vi "Get Magnet Field.vi"(6 "Axis":T1, 8 "error in (no error)":errorcluster, 11 "Instrument.Oxford1820 in":refnum<class "Instrument.Oxford1820.lvclass">) -> (0 "error out":errorcluster, 1 "Status":variant, 2 "B Field (T)":dbl, 3 "Instrument.Oxford1820 out":refnum<class "Instrument.Oxford1820.lvclass">, 4 "Finished?":bool)   [LabVIEW 2016, in "Instrument.Oxford1820.lvclass"]
uses:
  Instrument.Oxford1820.lvclass
  <userlib>/LevyLab/Levylab Instruments/Instrument Types/Cryostat/Typedefs/Magnet Axis--Enum.ctl
  Typedefs/Instrument.Oxford1820.Commands-enum.ctl
  <userlib>/LevyLab/Levylab Instruments/Instrument Types/Cryostat/Instrument.Cryostat.lvclass
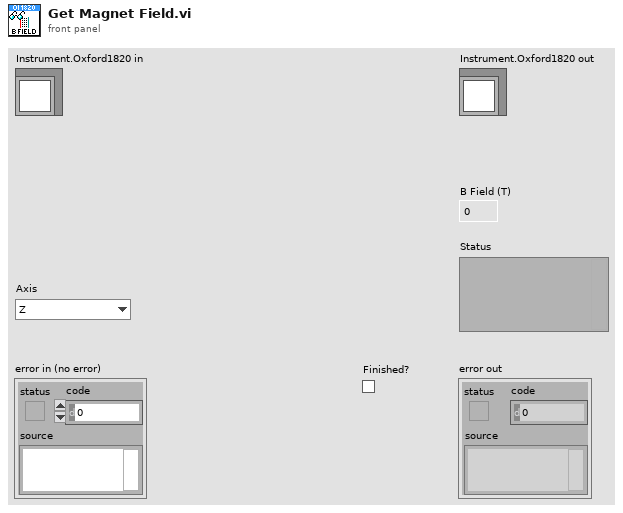
[diagram p1: front panel]
types:
  T1 = typedef "Instrument.Cryostat.lvclass/Magnet Axis--Enum.ctl" = enum16{"Z", "X", "Y"}
  T2 = typedef "Instrument.Oxford1820.lvclass/Instrument.Oxford1820.Commands-enum.ctl" = enum16{"setAction", "setTarget", "setSwitchHeat", "setLambda", "setFillMode", "setNeedleValve", "setMagnetField", "getStatus", "getTarget", "getSwitchHeat", "getPSUField", "newcommand", "getMagnetField"}
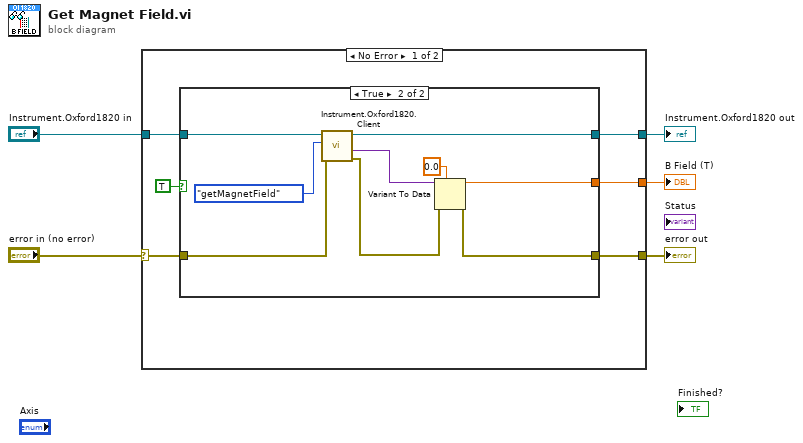
[diagram p0: block diagram]
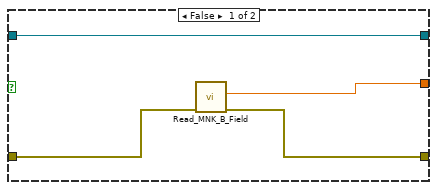
[diagram p2: hidden frame]
diagram:
  n1 = case shown="No Error" "error in (no error)" {
    selector: "error in (no error)" -> [w9 w26]
    tunnel: "Instrument.Oxford1820 in" -> [w7 w25]
    tunnel: [w11 w25] -> w4
    tunnel: [w10 _] -> w3
    tunnel: [w8 w26] -> w1
    frame No Error {
      n2 = case shown="True" TRUE {
        tunnel: [w12 w24] -> w11
        tunnel: [w13 w22] -> w10
        tunnel: w9 -> [w15 w21]
        tunnel: [w14 w20] -> w8
        tunnel: w7 -> [w12 w19]
        frame False {
          n3 = call "Read_MNK_B_Field.vi"("Read from DSC in"=w15) -> ("Read from DSC"=w14:errorcluster, "Field"=w13:dbl)  [unwired: 8 in, 1 out]
        }
        frame True {
          n4 = call "Instrument.Oxford1820.Client.vi"("error in (no error)"=w21, "Commands"=Instrument.Oxford1820.Commands-enum."getMagnetField", "Instrument.1820 in"=w19) -> ("error out"=w18:errorcluster, "Data out"=w17:variant, "Instrument.1820 out"=w24:refnum<class "Instrument.Oxford1820.lvclass">)  [unwired: 6 in]
          n5 = Variant To Data(error in=w18, type=0.0 ("B Field (T)"), Variant=w17) -> (data=w22:dbl, error out=w20:errorcluster)
        }
      }
    }
    frame Error {
    }
  }
  "error out" <- w1
  "Instrument.Oxford1820 out" <- w4
  "B Field (T)" <- w3
